vi "Edit Options.vi"(8 "error in (no error)":errorcluster, 10 "Calling VI in":refnum<vi>, 11 "Config":T1) -> (0 "error out":errorcluster, 2 "OK?":bool, 3 "Config out":T1)   [LabVIEW 2020, in "MacroAssert.lvlib"]
doc: "Displays a window to change any settings that have been established in the application."
uses:
  MacroAssert.lvlib
  FaKI State Machine/FaKI State Machine.lvlib
  a5ac09e5-38d3-43bc-9feb-68748838b8f7.vi
  CTLs/FGV Actions.ctl
  2b057859-5186-41e9-9ab4-790756e7a186.vi
  CTLs/Hotkey Type.ctl
  <vilib>/Utility/inputDevices.llb/keyboardAcquire.vi
  <vilib>/Utility/inputDevices.llb/closeKeyboard.vi
  CTLs/Config.ctl
panel:
  in  "OK":bool
  in  "Tab Control":enum32{"Reporting", "Hotkeys"}(tab)
  in  "Report Path":path
  in  "Save Report?":bool
  in  "Start/Stop":bool
  in  "Hotkey Type":T2
  out "Macro Hotkey":string
  out "Abort Hotkey":string
  in  "Exit":bool
  # "Change Hotkey\nPress Start Listening and hold down a key combination for five seconds to assign it as a hotkey."
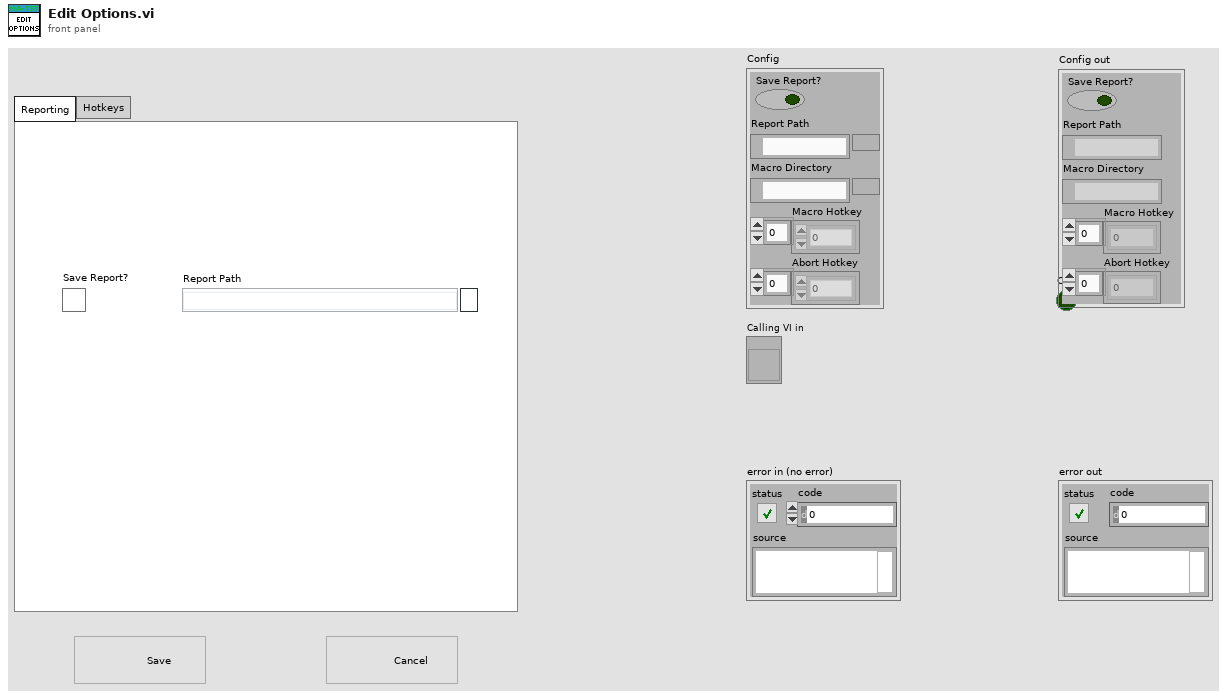
[diagram p1: front panel]
types:
  T1 = typedef "MacroAssert.lvlib/Config.ctl" = cluster{"Save Report?":bool, "Report Path":path, "Macro Directory":path, "Macro Hotkey":enum16{"0", "1", "2", "3", "4", "5", "6", "7", "8", "9", "A", "B", "C", "D", "E", "F", "G", "H", "I", "J", "K", "L", "M", "N", "O", "P", "Q", "R", "S", "T", "U", "V", "W", "X", "Y", "Z", "F1", "F2", "F3", "F4", "F5", "F6", "F7", "F8", "F9", "F10", "F11", "F12", "F13", "F14", "F15", "ADD", "BACK", "BACKSLASH", "CAPITAL", "COMMA", "DECIMAL", "DELETE", "DIVIDE", "DOWN", "END", "EQUALS", "ESCAPE", "GRAVE (`)", "HOME", "INSERT", "LBRACKET", "LCONTROL", "LEFT", "L ALT", "LSHIFT", "LWIN", "MINUS", "MULTIPLY", "NEXT", "NUMLOCK", "NUMPAD_0", "NUMPAD_1", "NUMPAD_2", "NUMPAD_3", "NUMPAD_4", "NUMPAD_5", "NUMPAD_6", "NUMPAD_7", "NUMPAD_8", "NUMPAD_9", "PAUSE", "PERIOD", "PRIOR (PG UP)", "RBRACKET", "RCONTROL", "RETURN", "RIGHT", "R ALT", "RSHIFT", "RWIN", "SCROLL", "SEMICOLON", "SLASH", "SPACE", "SUBTRACT", "TAB", "UP", "ENTER (num pad)", "' (quote)"}[], "Abort Hotkey":enum16{"0", "1", "2", "3", "4", "5", "6", "7", "8", "9", "A", "B", "C", "D", "E", "F", "G", "H", "I", "J", "K", "L", "M", "N", "O", "P", "Q", "R", "S", "T", "U", "V", "W", "X", "Y", "Z", "F1", "F2", "F3", "F4", "F5", "F6", "F7", "F8", "F9", "F10", "F11", "F12", "F13", "F14", "F15", "ADD", "BACK", "BACKSLASH", "CAPITAL", "COMMA", "DECIMAL", "DELETE", "DIVIDE", "DOWN", "END", "EQUALS", "ESCAPE", "GRAVE (`)", "HOME", "INSERT", "LBRACKET", "LCONTROL", "LEFT", "L ALT", "LSHIFT", "LWIN", "MINUS", "MULTIPLY", "NEXT", "NUMLOCK", "NUMPAD_0", "NUMPAD_1", "NUMPAD_2", "NUMPAD_3", "NUMPAD_4", "NUMPAD_5", "NUMPAD_6", "NUMPAD_7", "NUMPAD_8", "NUMPAD_9", "PAUSE", "PERIOD", "PRIOR (PG UP)", "RBRACKET", "RCONTROL", "RETURN", "RIGHT", "R ALT", "RSHIFT", "RWIN", "SCROLL", "SEMICOLON", "SLASH", "SPACE", "SUBTRACT", "TAB", "UP", "ENTER (num pad)", "' (quote)"}[]}
  T2 = typedef "MacroAssert.lvlib/Hotkey Type.ctl" = enum16{"Macro Hotkey", "Abort Hotkey"}
  T3 = enum32{"Invalid", "Standard", "Closed", "Hidden", "Minimized", "Maximized"}
  T4 = enum32{"invalid app kind", "Development System", "Run Time System", "Student Edition", "Embedded LabVIEW", "Evaluation", "Custom"}
  T5 = typedef "MacroAssert.lvlib/FGV Actions.ctl" = enum16{"Read", "Write"}
  T6 = cluster{"Core":cluster{"Current VI Reference":refnum<vi>, "Close Panel on Exit?":bool}, "Keyboard":refnum<k1>, "Last":enum16{"0", "1", "2", "3", "4", "5", "6", "7", "8", "9", "A", "B", "C", "D", "E", "F", "G", "H", "I", "J", "K", "L", "M", "N", "O", "P", "Q", "R", "S", "T", "U", "V", "W", "X", "Y", "Z", "F1", "F2", "F3", "F4", "F5", "F6", "F7", "F8", "F9", "F10", "F11", "F12", "F13", "F14", "F15", "ADD", "BACK", "BACKSLASH", "CAPITAL", "COMMA", "DECIMAL", "DELETE", "DIVIDE", "DOWN", "END", "EQUALS", "ESCAPE", "GRAVE (`)", "HOME", "INSERT", "LBRACKET", "LCONTROL", "LEFT", "L ALT", "LSHIFT", "LWIN", "MINUS", "MULTIPLY", "NEXT", "NUMLOCK", "NUMPAD_0", "NUMPAD_1", "NUMPAD_2", "NUMPAD_3", "NUMPAD_4", "NUMPAD_5", "NUMPAD_6", "NUMPAD_7", "NUMPAD_8", "NUMPAD_9", "PAUSE", "PERIOD", "PRIOR (PG UP)", "RBRACKET", "RCONTROL", "RETURN", "RIGHT", "R ALT", "RSHIFT", "RWIN", "SCROLL", "SEMICOLON", "SLASH", "SPACE", "SUBTRACT", "TAB", "UP", "ENTER (num pad)", "' (quote)"}[], "Config":T1, "OK?":bool}
  T7 = enum16{"0", "1", "2", "3", "4", "5", "6", "7", "8", "9", "A", "B", "C", "D", "E", "F", "G", "H", "I", "J", "K", "L", "M", "N", "O", "P", "Q", "R", "S", "T", "U", "V", "W", "X", "Y", "Z", "F1", "F2", "F3", "F4", "F5", "F6", "F7", "F8", "F9", "F10", "F11", "F12", "F13", "F14", "F15", "ADD", "BACK", "BACKSLASH", "CAPITAL", "COMMA", "DECIMAL", "DELETE", "DIVIDE", "DOWN", "END", "EQUALS", "ESCAPE", "GRAVE (`)", "HOME", "INSERT", "LBRACKET", "LCONTROL", "LEFT", "L ALT", "LSHIFT", "LWIN", "MINUS", "MULTIPLY", "NEXT", "NUMLOCK", "NUMPAD_0", "NUMPAD_1", "NUMPAD_2", "NUMPAD_3", "NUMPAD_4", "NUMPAD_5", "NUMPAD_6", "NUMPAD_7", "NUMPAD_8", "NUMPAD_9", "PAUSE", "PERIOD", "PRIOR (PG UP)", "RBRACKET", "RCONTROL", "RETURN", "RIGHT", "R ALT", "RSHIFT", "RWIN", "SCROLL", "SEMICOLON", "SLASH", "SPACE", "SUBTRACT", "TAB", "UP", "ENTER (num pad)", "' (quote)"}[]
  T8 = cluster{"Current VI Reference":refnum<vi>, "Close Panel on Exit?":bool}
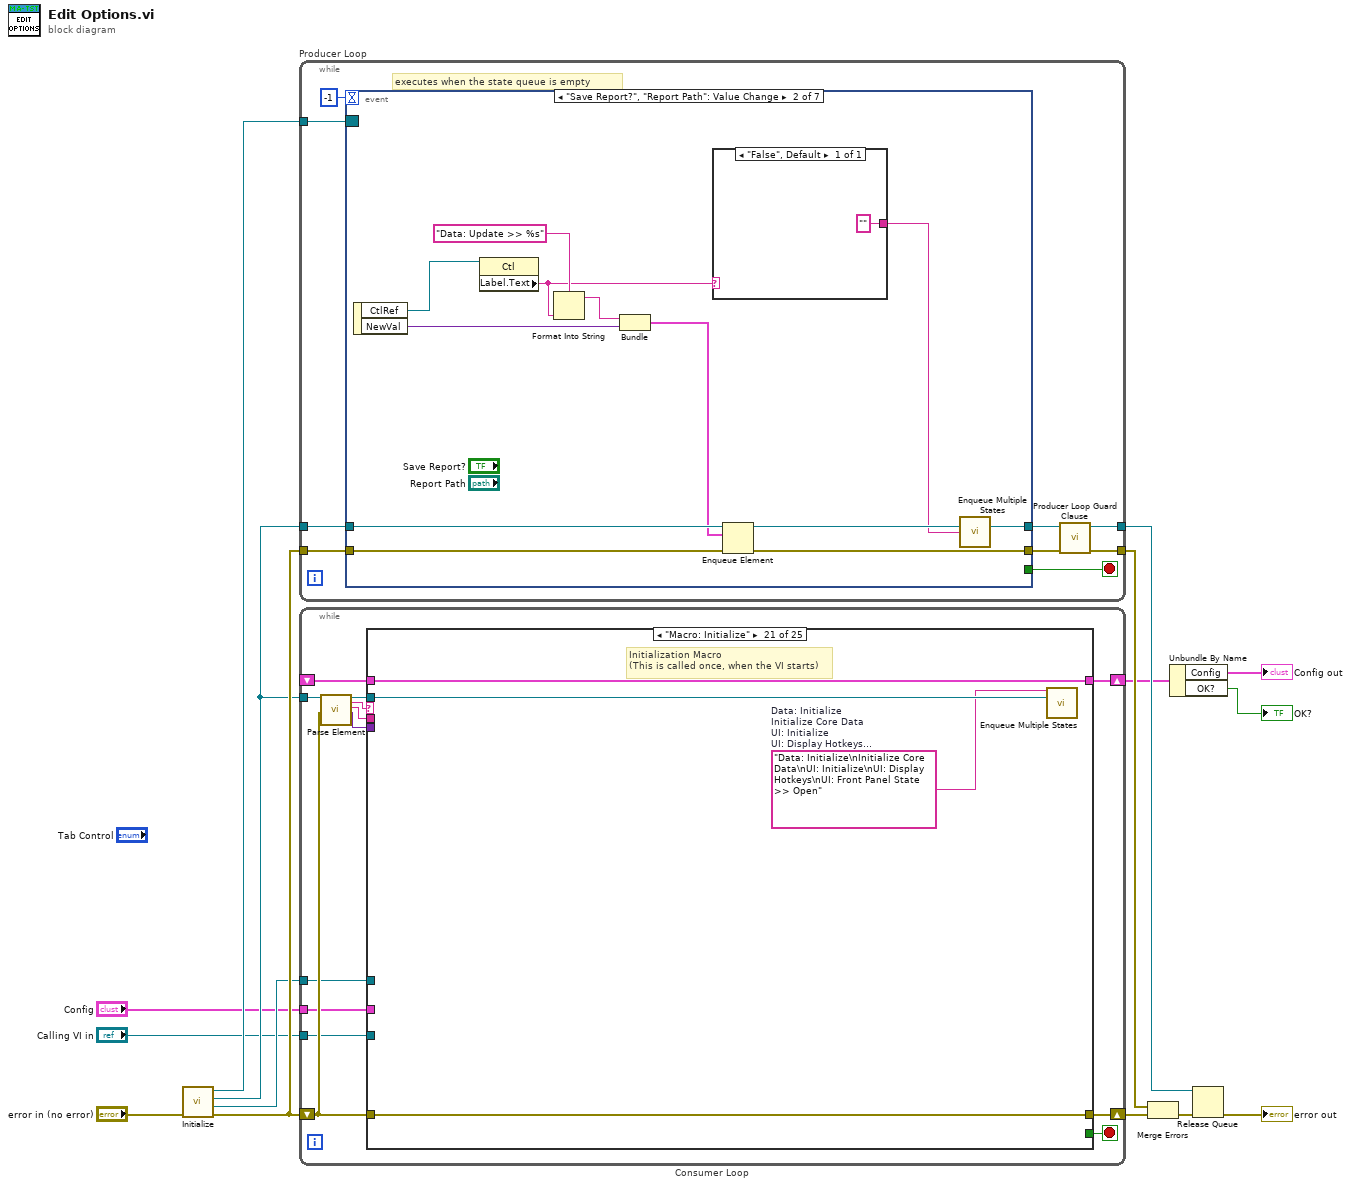
[diagram p0: block diagram]
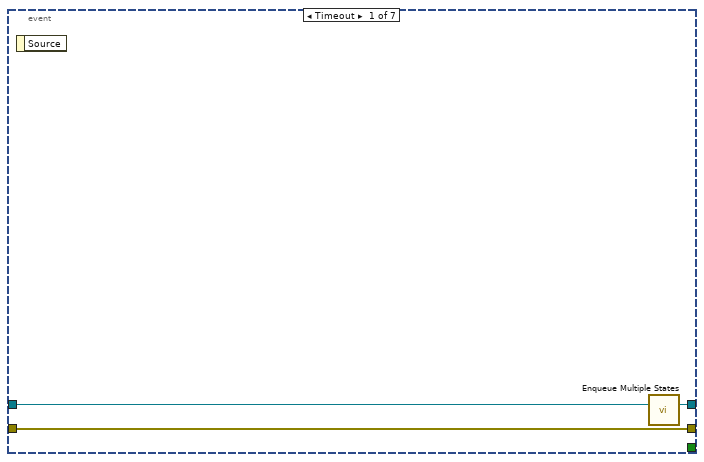
[diagram p2: hidden frame]
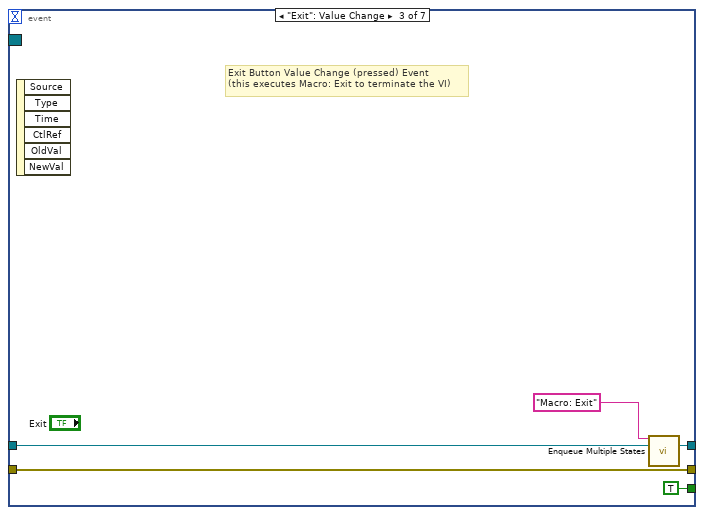
[diagram p3: hidden frame]
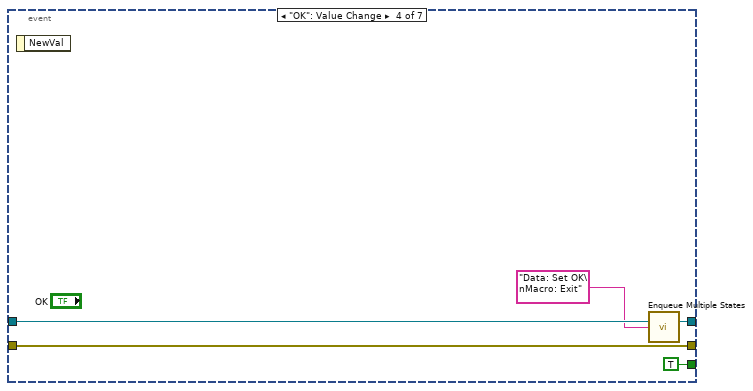
[diagram p4: hidden frame]
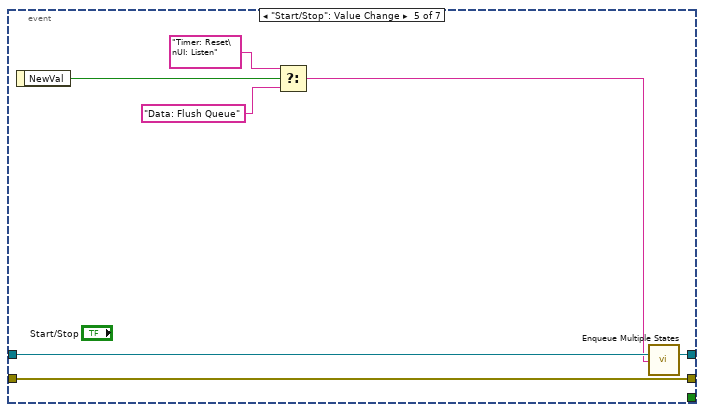
[diagram p5: hidden frame]
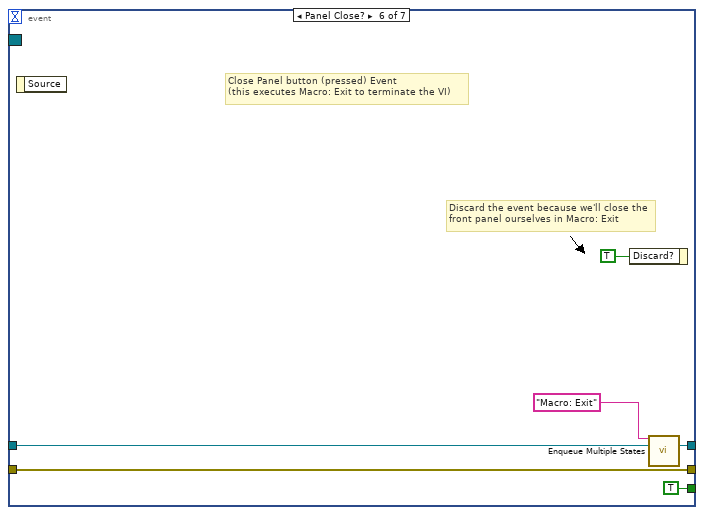
[diagram p6: hidden frame]
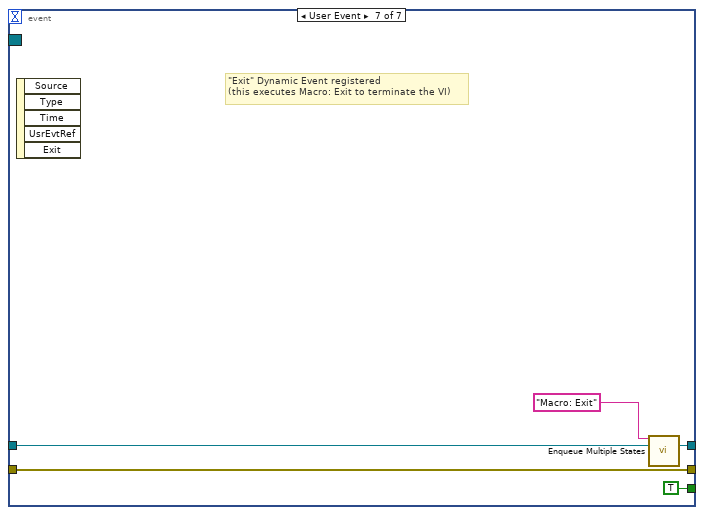
[diagram p7: hidden frame]
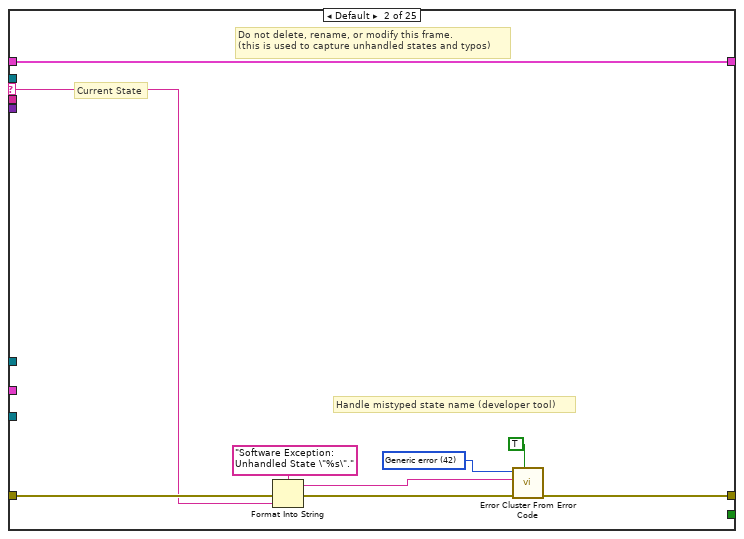
[diagram p9: hidden frame]
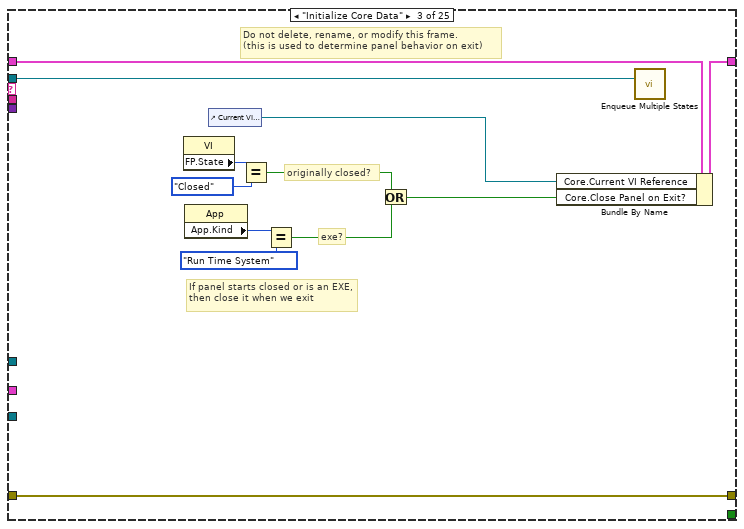
[diagram p10: hidden frame]
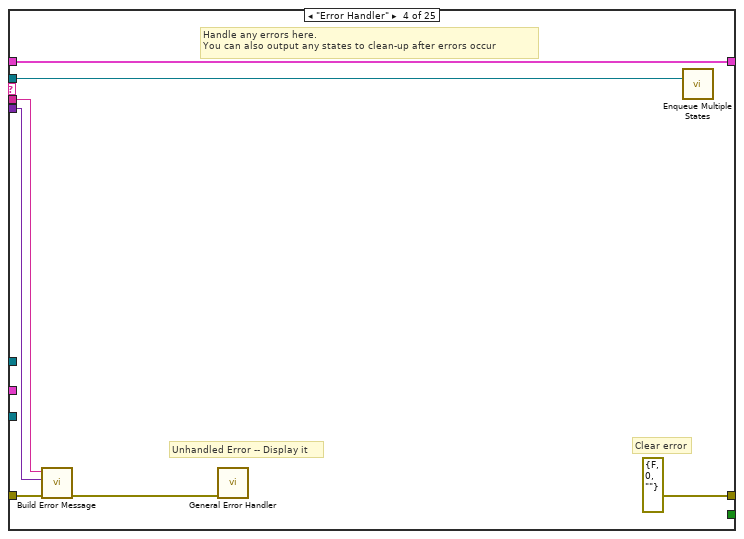
[diagram p11: hidden frame]
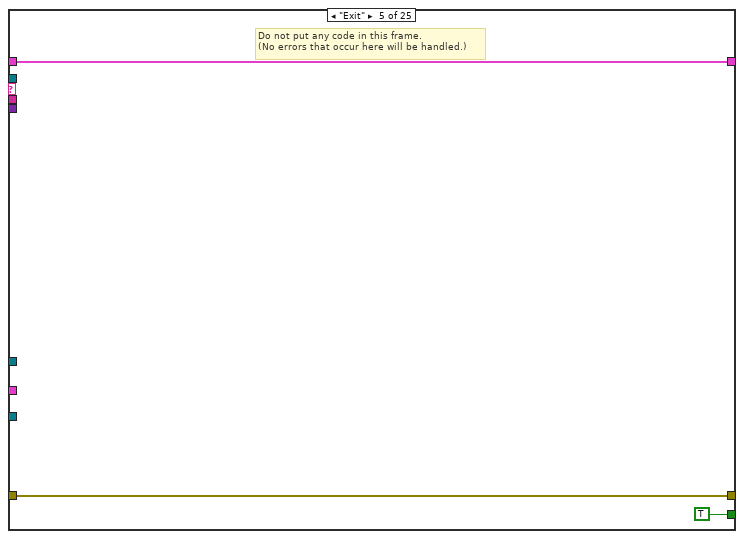
[diagram p12: hidden frame]
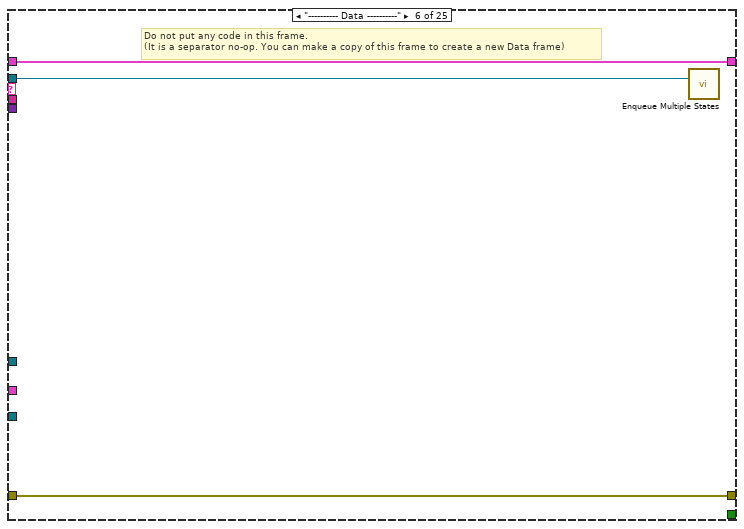
[diagram p13: hidden frame]
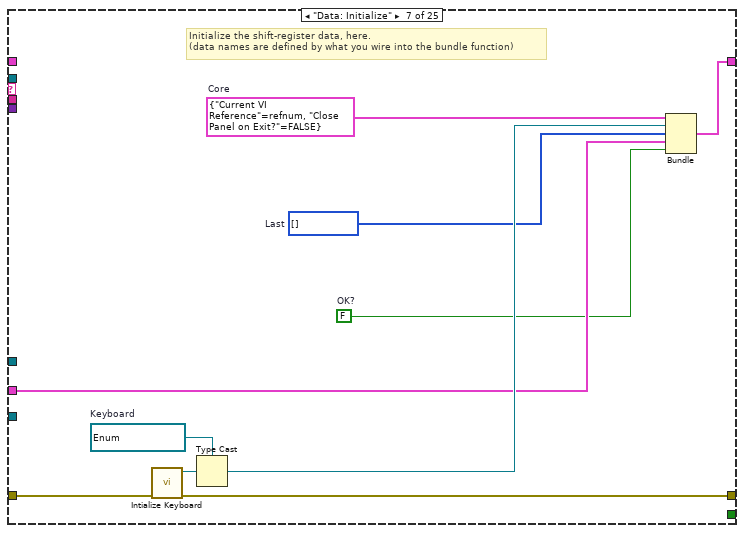
[diagram p14: hidden frame]
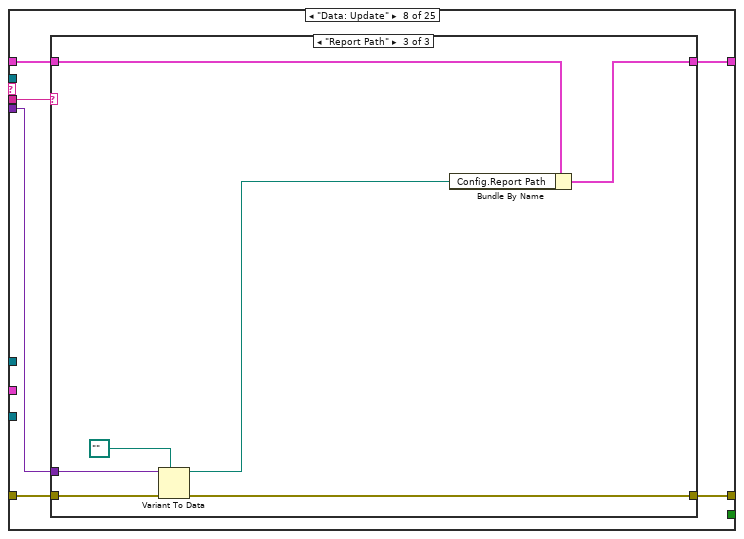
[diagram p15: hidden frame]
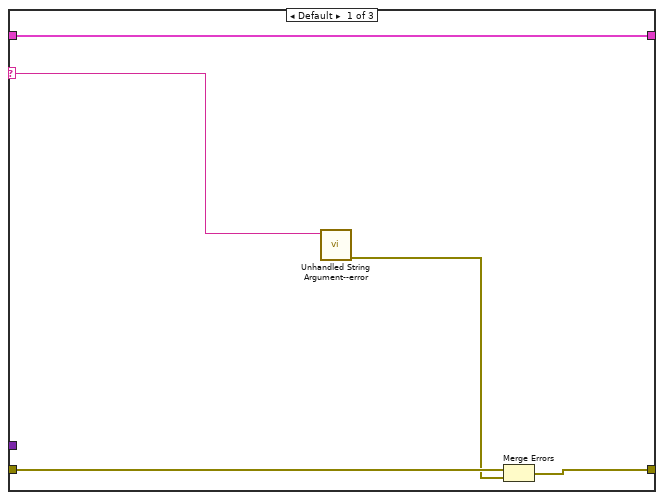
[diagram p16: hidden frame]
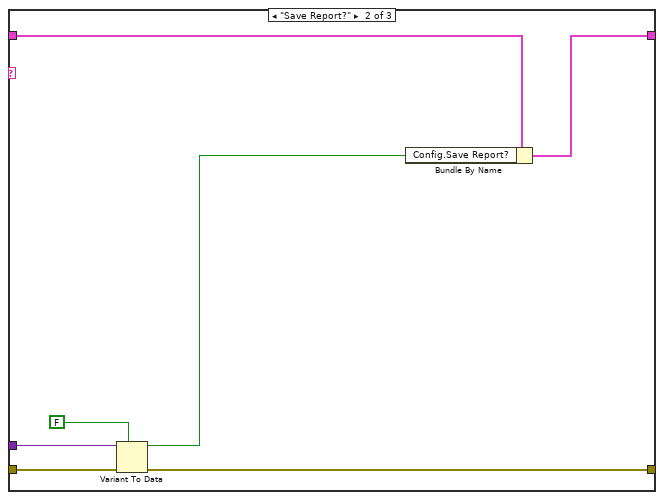
[diagram p17: hidden frame]
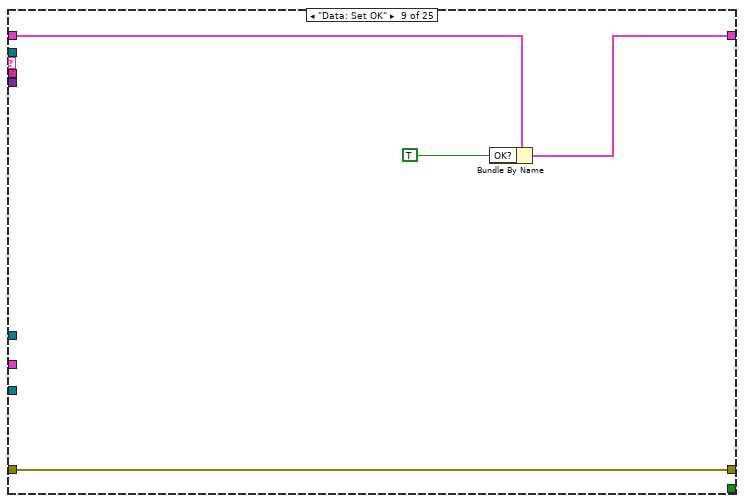
[diagram p18: hidden frame]
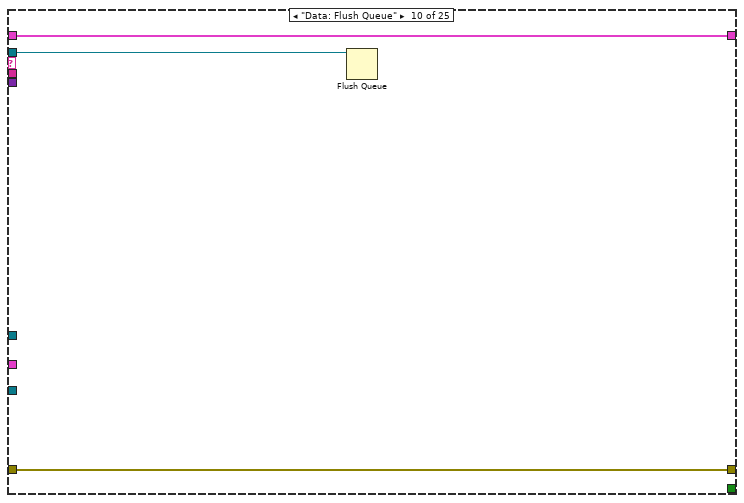
[diagram p19: hidden frame]
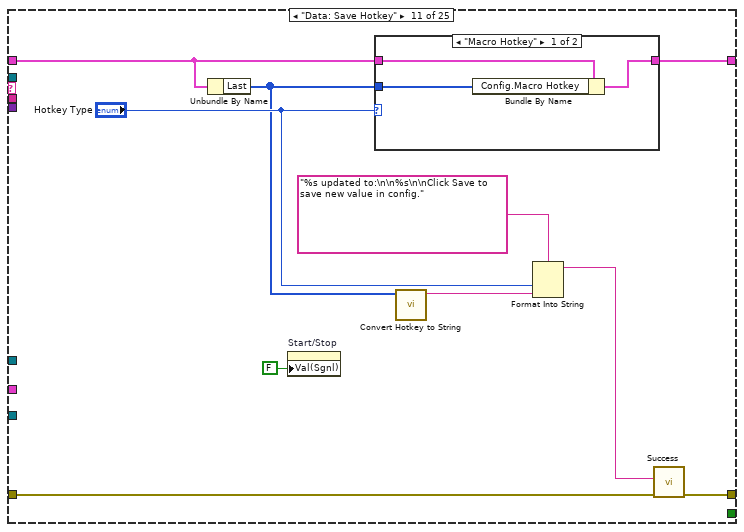
[diagram p20: hidden frame]
diagram:
  n1 = call "Initialize.vi"("error in (no error)"="error in (no error)") -> ("error out"=w10:errorcluster, "Exit Event"=w9:refnum<user-event>, "Queue"=w8:refnum<queue>, "Event Registration Refnum"=w7:refnum<event-registration>)  [unwired: 7 in]
  n2 = while "Producer Loop" {
    tunnel: w7 -> [w16]
    tunnel: w8 -> [w22]
    tunnel: [w17] -> w15
    tunnel: w10 -> [w24]
    tunnel: [w19] -> w13
    stop <- w21 stop-if-true
    # "executes when the state queue is empty"
    n3 = event shown="[1] \"Save Report?\", \"Report Path\": Value Change" {
      selector: w16 -> [_ _ _ _ _ _ _]
      dyn-events: _ -> [_ _ _ _ _ _ _]
      timeout: -1 ("Timeout") -> [_ _ _ _ _ _ _]
      tunnel: [w25 w31 w45 w50 w57 w63 w68] -> w20
      tunnel: w24 -> [w25 w32 w45 w50 w57 w63 w68]
      tunnel: w22 -> [w26 w39 w44 w49 w56 w60 w66]
      tunnel: [w27 w28 w42 w48 w55 w59 w65] -> w18
      tunnel: [_ _ TRUE TRUE _ TRUE TRUE] -> w21
      event Timeout {
        n4 = event-data() -> ()  [unwired: 1 in, 1 out]
        n5 = call "Enqueue Multiple States.vi"("queue in"=w26) -> ("queue out"=w27:refnum<queue>)  [unwired: 14 in]
      }
      event "Save Report?", "Report Path": Value Change {
        n6 = event-data() -> ("CtlRef"=w29:refnum<vi>, "NewVal"=w30:variant)  [unwired: 1 in]
        n7 = property class="Ctl"(reference=w29) -> ("Label.Text"=w34:string)  [unwired: 1 in, 2 out]
        n8 = Format Into String(format string="Data: Update >> %s", w34) -> (resulting string=w35:string)  [unwired: 2 in, 1 out]
        n9 = Bundle(w35, "NewVal"=w30) -> (w33:cluster{string, "NewVal":variant})  [unwired: 1 in]
        n10 = case shown="\"False\", Default" w34 {
          tunnel: ["" ("string")] -> w37
          frame "False", Default {
          }
        }
        n11 = Enqueue Element(queue=w39, element=w33, error in (no error)=w32) -> (queue out=w38:refnum<queue>, error out=w31:errorcluster)  [unwired: 1 in, 1 out]
        n12 = call "Enqueue Multiple States.vi"("queue in"=w38, "State(s) at Back"=w37) -> ("queue out"=w28:refnum<queue>)  [unwired: 13 in]
      }
      event "Exit": Value Change {
        # "Exit Button Value Change (pressed) Event\n(this executes Macro: Exit to terminate the VI)"
        n13 = event-data() -> ()  [unwired: 1 in, 6 out]
        n14 = call "Enqueue Multiple States.vi"("State(s) at Front"="Macro: Exit", "queue in"=w44) -> ("queue out"=w42:refnum<queue>)  [unwired: 13 in]
      }
      event "OK": Value Change {
        n15 = event-data() -> ()  [unwired: 1 in, 1 out]
        n16 = call "Enqueue Multiple States.vi"("queue in"=w49, "State(s) at Back"="Data: Set OK\nMacro: Exit") -> ("queue out"=w48:refnum<queue>)  [unwired: 13 in]
      }
      event "Start/Stop": Value Change {
        n17 = event-data() -> ("NewVal"=w54:bool)  [unwired: 1 in]
        n18 = Select(t="Timer: Reset\nUI: Listen", s=w54, f="Data: Flush Queue") -> (s? t:f=w51:string)
        n19 = call "Enqueue Multiple States.vi"("queue in"=w56, "State(s) at Back"=w51) -> ("queue out"=w55:refnum<queue>)  [unwired: 13 in]
      }
      event Panel Close? {
        # "Discard the event because we'll close the front panel ourselves in Macro: Exit"
        # "Close Panel button (pressed) Event\n(this executes Macro: Exit to terminate the VI)"
        n20 = event-data() -> ()  [unwired: 1 in, 1 out]
        n21 = event-data("Discard?"=TRUE) -> ()  [unwired: 1 in, 1 out]
        n22 = call "Enqueue Multiple States.vi"("State(s) at Front"="Macro: Exit", "queue in"=w60) -> ("queue out"=w59:refnum<queue>)  [unwired: 13 in]
      }
      event User Event {
        # "\"Exit\" Dynamic Event registered\n(this executes Macro: Exit to terminate the VI)"
        n23 = event-data() -> ()  [unwired: 1 in, 5 out]
        n24 = call "Enqueue Multiple States.vi"("State(s) at Front"="Macro: Exit", "queue in"=w66) -> ("queue out"=w65:refnum<queue>)  [unwired: 13 in]
      }
    }
    n25 = call "Producer Loop Guard Clause.vi"("error in (no error)"=w20, "queue in"=w18) -> ("error out"=w19:errorcluster, "queue out"=w17:refnum<queue>)  [unwired: 8 in]
  }
  n26 = while "Consumer Loop" {
    shift-right: [w78] -> w4
    shift-left: _ -> [w77]
    shift-right: [w81] -> w12
    shift-left: w10 -> [w80]
    tunnel: w8 -> [w76]
    tunnel: w9 -> [w71]
    tunnel: "Config" -> [w70]
    tunnel: "Calling VI in" -> [w69]
    stop <- w79 stop-if-true
    n27 = call "Parse Element.vi"("queue in"=w76, "error in (no error)"=w80) -> ("queue out"=w75:refnum<queue>, "State"=w74:string, "Arg"=w73:string, "Data"=w72:variant)  [unwired: 14 in]
    n28 = case shown="\"Macro: Initialize\"" w74 {
      selector: w74 -> [_ w84 _ _ _ _ _ _ _ _ _ _ _ _ _ _ _ _ _ _ _ _ _ _ _]
      tunnel: w75 -> [_ _ w93 w109 _ w115 _ _ _ w159 _ _ _ w187 w190 _ _ _ w294 _ w320 w327 _ _ w341]
      tunnel: w73 -> [_ _ _ w105 _ _ _ w133 _ _ _ _ _ _ _ w193 w202 _ _ _ _ _ _ _ _]
      tunnel: w77 -> [w82 w86 w99 w110 w113 w116 _ w132 w156 w158 w163 w179 w182 w184 w191 w194 w204 w276 w293 w317 w321 w331 w333 w339 w348]
      tunnel: [w83 w91 w104 errorcluster {"status"=FALSE, "code"=0, "source"=""} ("error out") w114 w117 w121 w129 w155 w157 w167 w177 w183 w188 w192 w195 w205 w277 w302 w318 w322 w332 w334 w337 w346] -> w81
      tunnel: w80 -> [w83 w90 w104 w108 w114 w117 w123 w131 w155 w157 w164 w181 w183 w188 w192 w196 w206 w277 w303 w318 w322 w332 w334 w338 w347]
      tunnel: [_ _ _ _ TRUE _ _ _ _ _ _ _ _ _ _ _ _ _ _ _ _ _ _ _ _] -> w79
      tunnel: [w82 w86 w103 w110 w113 w116 w127 w128 w154 w158 w161 w179 w182 w184 w191 w194 w204 w276 w292 w317 w321 w331 w333 w339 w348] -> w78
      tunnel: w72 -> [_ _ _ w106 _ _ _ w130 _ _ _ _ _ _ _ _ _ _ _ _ _ _ _ _ _]
      tunnel: w71 -> [_ _ _ _ _ _ _ _ _ _ _ _ _ _ _ _ _ _ _ _ _ _ _ _ _]
      tunnel: w70 -> [_ _ _ _ _ _ w119 _ _ _ _ _ _ _ _ _ _ _ _ _ _ _ _ _ _]
      tunnel: w69 -> [_ _ _ _ _ _ _ _ _ _ _ _ _ _ _ _ w201 _ _ _ _ _ _ _ _]
      frame "---------- Core ----------" {
        # "Do not put any code in this frame.\n(it is a separator no-op)"
      }
      frame Default {
        w88 = 42 items=["No error", "Argument error", "Memory is full", "Out of zone", "End of file", "File already open", "Generic file I/O error", "File not found", "File permission error", "Disk is full", "Duplicate path", "Too many files open", "System feature not enabled", "Resource file not found", "Cannot add resource", "Resource not found", "Image not found", "Image memory error", "Pen does not exist", "Config type invalid", "Config token not found", "Config parse error", "Config memory error", "Bad external code format", "Bad external code offset", "External code not present", "Null window", "Destroy window error", "Null menu", "Print aborted", "Bad print record", "Print driver error", "Windows error during printing", "Memory error during printing", "Print dialog error", "Generic print error", "Invalid device refnum", "Device not found", "Device parameter error", "Device unit error", "Cannot open device", "Device call aborted", "Generic error", "Cancelled by user", "Object ID too low", "Object ID too high", "Object not in heap", "Unknown heap", "Unknown object (invalid DefProc)", "Unknown object (DefProc not in table)", "Message out of range", "Invalid (null) method", "Unknown message", "Manager call not supported", "Bad address", "Network operation in progress", "Network operation timed out", "Connection is busy", "Network attribute not supported", "Network error", "Address in use", "System out of memory", "Connection aborted", "Connection refused", "Not connected", "Already connected", "Connection closed", "Initialization error (interapplication manager)", "Bad occurrence", "Wait on unbound occurrence handler", "Occurrence queue overflow", "Datalog type conflict", "Unused", "Unrecognized type (interapplication manager)", "Memory corrupt", "Failed to make temporary DLL", "Old CIN version", "Drag socket not found", "Failed to load drop-object", "Failed to register OLE object", "Failed to release OLE object", "Format specifier type mismatch", "Unknown format specifier", "Too few format specifiers", "Too many format specifiers", "Scan failed", "Newer CIN version", "Error converting to variant", "Runtime menu error", "Password tampered", "Variant attribute not found", "Incompatible variant data type", "Event data is not available", "Event Store is not present", "Occurrence is not found", "Event Queue is not created", "Event info is not available", "Refnum passed is NULL", "Error retrieving Class GUID", "Error retrieving CoClass GUID", "Error retrieving TypeLib GUID.", "Bad built application magic bytes.", "Specific driver is different from the specific driver associated with the Logical Name.", "There is no session opened to the class driver.", "Max Error", "MAX - Error with config objects", "MAX - Error loading configuration", "MAX - Group not supported"]
        # "Current State"
        # "Do not delete, rename, or modify this frame.\n(this is used to capture unhandled states and typos)"
        # "Handle mistyped state name (developer tool)"
        n29 = Format Into String(format string="Software Exception: Unhandled State \"%s\"." ("message"), error in=w90, w84) -> (resulting string=w87:string, error out=w92:errorcluster)  [unwired: 1 in]
        n30 = call <vilib>:"Error Cluster From Error Code.vi"("show call chain? (False)"=TRUE, "error in (no error)"=w92, "error message (\"\")"=w87, "error code (0)"=w88) -> ("error out"=w91:errorcluster)  [unwired: 5 in]
      }
      frame "Initialize Core Data" {
        # "Do not delete, rename, or modify this frame.\n(this is used to determine panel behavior on exit)"
        # "originally closed?"
        # "exe?"
        # "If panel starts closed or is an EXE, then close it when we exit"
        n31 = property class="VI"() -> ("FP.State"=w96:T3)  [unwired: 2 in, 2 out]
        n32 = property class="App"() -> ("App.Kind"=w102:T4)  [unwired: 2 in, 2 out]
        n33 = control-ref of="Current VI Reference"() -> (w97:refnum<vi>)
        n34 = Equal?(x=w96, y=T3."Closed" ("Front Panel Window:State")) -> (x = y?=w94:bool)
        n35 = Equal?(x=w102, y=T4."Run Time System" ("Application:Kind")) -> (x = y?=w100:bool)
        n36 = Or(x=w94, y=w100) -> (x .or. y?=w98:bool)
        n37 = Bundle By Name(cluster=w99, "Core.Current VI Reference"=w97, "Core.Close Panel on Exit?"=w98) -> (w103:T6)
        n38 = call "Enqueue Multiple States.vi"("queue in"=w93) -> ()  [unwired: 14 in, 1 out]
      }
      frame "Error Handler" {
        # "Unhandled Error -- Display it"
        # "Handle any errors here.\nYou can also output any states to clean-up after errors occur"
        # "Clear error"
        n39 = call "Build Error Message.vi"("error in (no error)"=w108, "Data"=w106, "Arg"=w105) -> ("error out"=w107:errorcluster)  [unwired: 8 in]
        n40 = call <vilib>:"General Error Handler.vi"("error in (no error)"=w107) -> ()  [unwired: 10 in, 5 out]
        n41 = call "Enqueue Multiple States.vi"("queue in"=w109) -> ()  [unwired: 14 in, 1 out]
      }
      frame "Exit" {
        # "Do not put any code in this frame.\n(No errors that occur here will be handled.)"
      }
      frame "---------- Data ----------" {
        # "Do not put any code in this frame.\n(It is a separator no-op. You can make a copy of this frame to create a new Data frame)"
        n42 = call "Enqueue Multiple States.vi"("queue in"=w115) -> ()  [unwired: 14 in, 1 out]
      }
      frame "Data: Initialize" {
        w118 = FALSE  # OK?
        w120 = T7 [] items=["0", "1", "2", "3", "4", "5", "6", "7", "8", "9", "A", "B", "C", "D", "E", "F", "G", "H", "I", "J", "K", "L", "M", "N", "O", "P", "Q", "R", "S", "T", "U", "V", "W", "X", "Y", "Z", "F1", "F2", "F3", "F4", "F5", "F6", "F7", "F8", "F9", "F10", "F11", "F12", "F13", "F14", "F15", "ADD", "BACK", "BACKSLASH", "CAPITAL", "COMMA", "DECIMAL", "DELETE", "DIVIDE", "DOWN", "END", "EQUALS", "ESCAPE", "GRAVE (`)", "HOME", "INSERT", "LBRACKET", "LCONTROL", "LEFT", "L ALT", "LSHIFT", "LWIN", "MINUS", "MULTIPLY", "NEXT", "NUMLOCK", "NUMPAD_0", "NUMPAD_1", "NUMPAD_2", "NUMPAD_3", "NUMPAD_4", "NUMPAD_5", "NUMPAD_6", "NUMPAD_7", "NUMPAD_8", "NUMPAD_9", "PAUSE", "PERIOD", "PRIOR (PG UP)", "RBRACKET", "RCONTROL", "RETURN", "RIGHT", "R ALT", "RSHIFT", "RWIN", "SCROLL", "SEMICOLON", "SLASH", "SPACE", "SUBTRACT", "TAB", "UP", "ENTER (num pad)", "' (quote)"]  # Last
        w124 = refnum<k1> refnum items=["KEYBOARD"]  # Keyboard
        w126 = T8 {"Current VI Reference"=refnum, "Close Panel on Exit?"=FALSE}  # Core
        # "Initialize the shift-register data, here.\n(data names are defined by what you wire into the bundle function)"
        n43 = call <vilib>:"Intialize Keyboard.vi"("error in (no error)"=w123) -> ("error out"=w121:errorcluster, "device ID"=w125:refnum<k1>)  [unwired: 9 in]
        n44 = Type Cast(type=w124, x=w125) -> (*(type *) &x=w122:refnum<k1>)
        n45 = Bundle("Core"=w126, "Keyboard"=w122, "Last"=w120, "Config"=w119, "OK?"=w118) -> (w127:T6)  [unwired: 1 in]
      }
      frame "Data: Update" {
        n46 = case shown="\"Report Path\"" w133 {
          selector: w133 -> [w136 _ _]
          tunnel: w132 -> [w134 w145 w152]
          tunnel: w131 -> [w138 w144 w151]
          tunnel: w130 -> [_ w143 w150]
          tunnel: [w135 w141 w148] -> w129
          tunnel: [w134 w139 w146] -> w128
          frame Default {
            n47 = call "Unhandled String Argument--error.vi"("Argument"=w136) -> ("error out"=w137:errorcluster)  [unwired: 10 in]
            n48 = Merge Errors(w138, w137) -> (w135:errorcluster)
          }
          frame "Save Report?" {
            n49 = Variant To Data(error in=w144, type=FALSE, Variant=w143) -> (data=w140:bool, error out=w141:errorcluster)
            n50 = Bundle By Name(cluster=w145, "Config.Save Report?"=w140) -> (w139:T6)
          }
          frame "Report Path" {
            n51 = Variant To Data(error in=w151, type=path "", Variant=w150) -> (data=w147:path, error out=w148:errorcluster)
            n52 = Bundle By Name(cluster=w152, "Config.Report Path"=w147) -> (w146:T6)
          }
        }
      }
      frame "Data: Set OK" {
        n53 = Bundle By Name(cluster=w156, "OK?"=TRUE) -> (w154:T6)
      }
      frame "Data: Flush Queue" {
        n54 = Flush Queue(queue=w159) -> ()  [unwired: 1 in, 3 out]
      }
      frame "Data: Save Hotkey" {
        n55 = Unbundle By Name(w163) -> ("Last"=w160:T7)
        n56 = property on="Start/Stop" class="Bool (strict)"("Val(Sgnl)"=FALSE ("Value (Signaling)")) -> ()  [unwired: 2 in, 2 out]
        n57 = case shown="\"Macro Hotkey\"" "Hotkey Type" {
          tunnel: w163 -> [w172 w175]
          tunnel: [w171 w174] -> w161
          tunnel: w160 -> [w170 w173]
          frame "Macro Hotkey" {
            n58 = Bundle By Name(cluster=w172, "Config.Macro Hotkey"=w170) -> (w171:T6)
          }
          frame "Abort Hotkey" {
            n59 = Bundle By Name(cluster=w175, "Config.Abort Hotkey"=w173) -> (w174:T6)
          }
        }
        n60 = call "Convert Hotkey to String.vi"("Hotkey"=w160) -> ("String"=w165:string)  [unwired: 10 in]
        n61 = Format Into String(format string="%s updated to:\n\n%s\n\nClick Save to save new value in config.", "Hotkey Type", w165) -> (resulting string=w168:string)  [unwired: 2 in, 1 out]
        n62 = call "Success"("error in (no error)"=w164, "Message"=w168) -> ("error out"=w167:errorcluster)  [unwired: 8 in, 1 out]
      }
      frame "Data: Cleanup" {
        # "Cleanup any data and references, here.\n(this is called automatically, by the Macro: Exit)"
        n63 = Unbundle By Name(w179) -> ("Core.Current VI Reference"=w180:refnum<vi>, "Keyboard"=w176:refnum<k1>)
        n64 = Close Reference(reference=w180, error in (no error)=w181) -> (error out=w178:errorcluster)
        n65 = call-poly <vilib>:"Close Input Device.vi"("error in (no error)"=w178, "device ID"=w176) -> ("error out"=w177:errorcluster)  [unwired: 8 in]
      }
      frame "---------- UI ----------" {
        # "Do not put any code in this frame.\n(It is a separator no-op. You can make a copy of this frame to create a new UI frame)"
      }
      frame "UI: Initialize" {
        # "Initialize the User Interface, here.\n(this is called automatically, by the Macro: Init)"
        n66 = Unbundle By Name(w184) -> ("Config.Save Report?"=w186:bool, "Config.Report Path"=w185:path)
        n67 = local write "Save Report?"(w186) -> ()
        n68 = local write "Report Path"(w185) -> ()
        n69 = call "Enqueue Multiple States.vi"("queue in"=w187) -> ()  [unwired: 14 in, 1 out]
      }
      frame "UI: Uninitialize" {
        # "Uninitialize the User Interface, here.\n(this is called automatically, by the Macro: Exit)"
        n70 = property on="Tab Control" class="TabCtl (strict)"("Value"=enum32{"Reporting", "Hotkeys"}."Reporting" ("Tab Control")) -> ()  [unwired: 2 in, 2 out]
        n71 = call "Enqueue Multiple States.vi"("queue in"=w190) -> ()  [unwired: 14 in, 1 out]
      }
      frame "UI: Cursor Set" {
        # "Argument"
        # "Set and Unset Cursor Busy.\n(Usage: \"UI: Cursor Set >> Busy|Idle\")"
        n72 = case shown="\"Idle\", Default" w193 {
          tunnel: w196 -> [w198 w200]
          tunnel: [w197 w199] -> w195
          frame "Idle", Default {
            n73 = call <vilib>:"Unset Busy.vi"("error in (no error)"=w198) -> ("error out"=w197:errorcluster)  [unwired: 10 in]
          }
          frame "Busy" {
            n74 = call <vilib>:"Set Busy.vi"("error in (no error)"=w200) -> ("error out"=w199:errorcluster)  [unwired: 9 in, 1 out]
          }
        }
      }
      frame "UI: Front Panel State" {
        # "Argument"
        # "Set Front Panel Open or Closed\n(Usage: \"UI: Front Panel State >> Open|Close\")"
        n75 = Unbundle By Name(w204) -> ("Core.Current VI Reference"=w203:refnum<vi>)
        n76 = case shown="\"Open\", \"Standard\", Default" w202 {
          tunnel: w206 -> [w214 w231 w243 w256 w269]
          tunnel: [w215 w232 w244 w257 w270] -> w205
          tunnel: w203 -> [w212 w229 w241 w254 w267]
          tunnel: w201 -> [w207 _ _ _ _]
          frame "Open", "Standard", Default {
            w208 = T3."Standard" ("State")
            n77 = property class="VI"(reference=w212, error in=w214) -> (reference out=w211:refnum<vi>, error out=w213:errorcluster, "FP.State"=w210:T3)
            n78 = Not Equal?(x=w210, y=w208) -> (x != y?=w209:bool)
            n79 = case shown="True" w209 {
              tunnel: [w223 w224] -> w215
              tunnel: w213 -> [w220 w224]
              tunnel: w211 -> [w219 _]
              tunnel: w208 -> [w221 _]
              tunnel: w207 -> [w216 _]
              frame True {
                n80 = call "Center Dialog on Caller.vi"("error in (no error)"=w220, "Dialog VI"=w219, "Calling VI in"=w216) -> ("error out"=w218:errorcluster, "Dialog VI out"=w217:refnum<vi>)  [unwired: 7 in]
                n81 = invoke class="VI" method="FP.Open"(reference=w217, error in=w218, "Activate"=TRUE, "State"=w221) -> (error out=w223:errorcluster)  [unwired: 1 in, 4 out]
              }
              frame False {
              }
            }
          }
          frame "Close", "Closed" {
            n82 = property class="VI"(reference=w229, error in=w231) -> (reference out=w228:refnum<vi>, error out=w230:errorcluster, "FP.State"=w226:T3)
            n83 = Not Equal?(x=w226, y=T3."Closed" ("Front Panel Window:State")) -> (x != y?=w225:bool)
            n84 = case shown="True" w225 {
              tunnel: [w233 w236] -> w232
              tunnel: w230 -> [w233 w235]
              tunnel: w228 -> [_ w234]
              frame False {
              }
              frame True {
                n85 = invoke class="VI" method="FP.Close"(reference=w234, error in=w235) -> (error out=w236:errorcluster)  [unwired: 1 in, 2 out]
              }
            }
          }
          frame "Hidden", "Hide" {
            w237 = T3."Hidden" ("State")
            n86 = property class="VI"(reference=w241, error in=w243) -> (reference out=w240:refnum<vi>, error out=w242:errorcluster, "FP.State"=w239:T3)
            n87 = Not Equal?(x=w239, y=w237) -> (x != y?=w238:bool)
            n88 = case shown="True" w238 {
              tunnel: [w248 w249] -> w244
              tunnel: w242 -> [w247 w249]
              tunnel: w240 -> [w246 _]
              tunnel: w237 -> [w245 _]
              frame True {
                n89 = invoke class="VI" method="FP.Open"(reference=w246, error in=w247, "State"=w245) -> (error out=w248:errorcluster)  [unwired: 2 in, 4 out]
              }
              frame False {
              }
            }
          }
          frame "Minimize", "Minimized" {
            w250 = T3."Minimized" ("State")
            n90 = property class="VI"(reference=w254, error in=w256) -> (reference out=w253:refnum<vi>, error out=w255:errorcluster, "FP.State"=w252:T3)
            n91 = Not Equal?(x=w252, y=w250) -> (x != y?=w251:bool)
            n92 = case shown="True" w251 {
              tunnel: [w261 w262] -> w257
              tunnel: w255 -> [w260 w262]
              tunnel: w253 -> [w259 _]
              tunnel: w250 -> [w258 _]
              frame True {
                n93 = invoke class="VI" method="FP.Open"(reference=w259, error in=w260, "State"=w258) -> (error out=w261:errorcluster)  [unwired: 2 in, 4 out]
              }
              frame False {
              }
            }
          }
          frame "Maximize", "Maximized" {
            w263 = T3."Maximized" ("State")
            n94 = property class="VI"(reference=w267, error in=w269) -> (reference out=w266:refnum<vi>, error out=w268:errorcluster, "FP.State"=w265:T3)
            n95 = Not Equal?(x=w265, y=w263) -> (x != y?=w264:bool)
            n96 = case shown="True" w264 {
              tunnel: [w274 w275] -> w270
              tunnel: w268 -> [w273 w275]
              tunnel: w266 -> [w272 _]
              tunnel: w263 -> [w271 _]
              frame True {
                n97 = invoke class="VI" method="FP.Open"(reference=w272, error in=w273, "State"=w271) -> (error out=w274:errorcluster)  [unwired: 2 in, 4 out]
              }
              frame False {
              }
            }
          }
        }
      }
      frame "UI: Display Hotkeys" {
        n98 = Unbundle By Name(w276) -> ("Config.Macro Hotkey"=w280:T7, "Config.Abort Hotkey"=w278:T7)
        n99 = call "Convert Hotkey to String.vi"("Hotkey"=w280) -> ("String"=→"Macro Hotkey":string)  [unwired: 10 in]
        n100 = call "Convert Hotkey to String.vi"("Hotkey"=w278) -> ("String"=→"Abort Hotkey":string)  [unwired: 10 in]
      }
      frame "UI: Listen" {
        # "#TODO refactor, add interlocks to prevent OK/cancel button press while listening"
        n101 = Unbundle By Name(w293) -> ("Config"=w288:T1, "Last"=w300:T7, "Keyboard"=w307:refnum<k1>)
        n102 = call "Stall Data Flow.vim"("value in"=w307, "milliseconds to wait"=u32 1) -> ("value out"=w305:refnum<k1>)  [unwired: 1 out]
        n103 = Empty Array?(array=w300) -> (empty?=w301:bool)
        n104 = call-poly <vilib>:"Acquire Input Data.vi"("device ID"=w305, "error in (no error)"=w303) -> ("keys pressed"=w306:T7, "error out"=w302:errorcluster)  [unwired: 15 in, 1 out]
        n105 = call "Enum to Array of Enums.vim"("enum"=Hotkey_Type."Macro Hotkey" ("Hotkey Type")) -> ("array of enums"=w290:T2[])
        n106 = Not(x=w301) -> (.not. x?=w298:bool)
        n107 = Sort 1D Array(array=w306) -> (sorted array=w287:T7)
        n108 = Equal?(x=w300, y=w287) -> (x = y?=w299:bool)
        n109 = for {
          tunnel: w290 -> [w311] mode=indexing
          tunnel: w288 -> [w312]
          tunnel: [w311] -> w285 if=w308
          tunnel: w287 -> [w310]
          tunnel: [w308] -> w283
          stop <- w308 stop-if-true
          n110 = case shown="\"Abort Hotkey\"" w311 {
            tunnel: w312 -> [w314 w316]
            tunnel: [w313 w315] -> w309
            frame "Macro Hotkey", Default {
              n111 = Unbundle By Name(w314) -> ("Macro Hotkey"=w313:T7)
            }
            frame "Abort Hotkey" {
              n112 = Unbundle By Name(w316) -> ("Abort Hotkey"=w315:T7)
            }
          }
          n113 = Equal?(x=w309, y=w310) -> (x = y?=w308:bool)
        }
        n114 = Not(x=w283) -> (.not. x?=w282:bool)
        n115 = Format Into String(format string="That key combination is already assigned as the %s.", w285) -> (resulting string=w284:string)  [unwired: 2 in, 1 out]
        n116 = Compound Arithmetic op=AND(w282, w298, w299) -> (w297:bool)
        n117 = call "Already Assigned"("Enable"=w283, "Message"=w284) -> ()  [unwired: 8 in, 2 out]
        n118 = Select(t="Timer: Poll", s=w297, f="Timer: Reset\nUI: Listen") -> (s? t:f=w291:string)
        n119 = call "Enqueue Multiple States.vi"("queue in"=w294, "State(s) at Back"=w291) -> ()  [unwired: 13 in, 1 out]
        n120 = Bundle By Name(cluster=w293, "Last"=w287) -> (w292:T6)
      }
      frame "---------- Macro ----------" {
        # "Do not put any code in this frame.\n(It is a separator no-op. You can make a copy of this frame to create a new Macro frame)"
      }
      frame "Macro: Initialize" {
        w319 = "Data: Initialize\nInitialize Core Data\nUI: Initialize\nUI: Display Hotkeys\nUI: Front Panel State >> Open"  # Data: Initialize Initialize Core Data UI: Initialize UI: Display Hotkeys UI: Front Panel State >> Open
        # "Initialization Macro\n(This is called once, when the VI starts)"
        n121 = call "Enqueue Multiple States.vi"("State(s) at Front"=w319, "queue in"=w320) -> ()  [unwired: 13 in, 1 out]
      }
      frame "Macro: Exit" {
        # "Exit Macro\n(This is called once, when the VI exits)"
        n122 = Unbundle By Name(w331) -> ("Core.Close Panel on Exit?"=w330:bool)
        n123 = Select(t="UI: Front Panel State >> Close\n", s=w330, f="") -> (s? t:f=w326:string)
        n124 = Concatenate Strings("UI: Uninitialize\n", w326, "Data: Cleanup\nExit") -> (w324:string)
        n125 = call "Enqueue Multiple States.vi"("State(s) at Front"=w324, "queue in"=w327) -> ()  [unwired: 13 in, 1 out]
      }
      frame "---------- Timer ----------" {
        # "Template Separator\n(You can make a copy of, or modify, this frame)"
      }
      frame "Timer: Reset" {
        n126 = call "Timer FGV.vi"("Mode"=FGV_Actions."Write", "error in (no error)"=w338, "Timer Value (s)"=5.0) -> ("error out"=w337:errorcluster)  [unwired: 6 in, 2 out]
      }
      frame "Timer: Poll" {
        n127 = call "Timer FGV.vi"("Mode"=FGV_Actions."Read", "error in (no error)"=w347) -> ("error out"=w346:errorcluster, "Expired?"=w344:bool)  [unwired: 7 in, 1 out]
        n128 = Select(t="Data: Save Hotkey\nUI: Display Hotkeys", s=w344, f="UI: Listen") -> (s? t:f=w340:string)
        n129 = call "Enqueue Multiple States.vi"("queue in"=w341, "State(s) at Back"=w340) -> ()  [unwired: 13 in, 1 out]
      }
    }
  }
  n130 = Merge Errors(w13, w12) -> (w14:errorcluster)
  n131 = Unbundle By Name(w4) -> ("Config"=→"Config out":T1, "OK?"=→"OK?":bool)
  n132 = Release Queue(queue=w15, error in (no error)=w14) -> (error out=→"error out":errorcluster)  [unwired: 1 in, 2 out]
